vi "Set acquisition mode.vi"(8 "Error In":errorcluster, 9 "Synchronous acquisition":bool, 11 "Camera reference in":refnum<k24>) -> (0 "Error Out":errorcluster, 3 "Camera reference out":refnum<k24>)   [LabVIEW 2017]
uses:
  C:/Program Files/National Instruments/LabVIEW 2017/instr.lib/IDS/ueye.NET/uEyeDotNet.dll
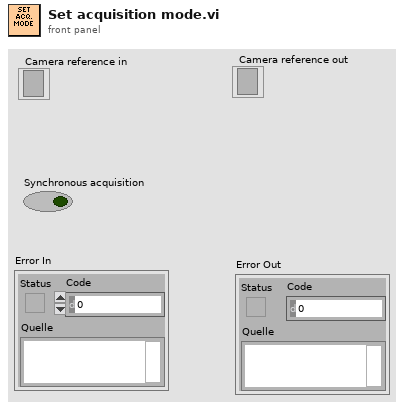
[diagram p1: front panel]
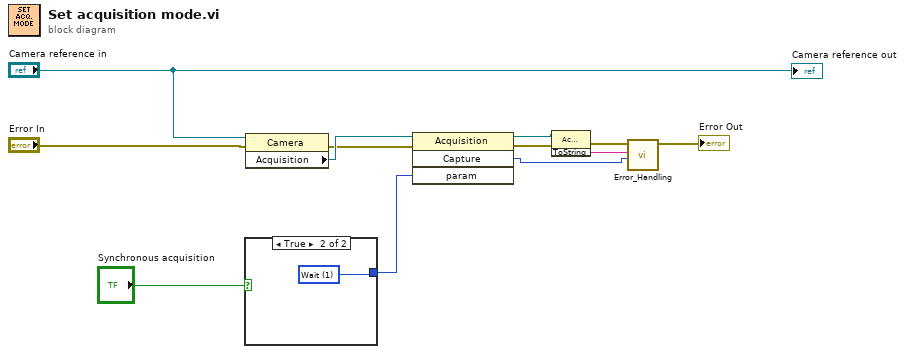
[diagram p0: block diagram]
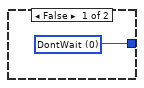
[diagram p2: hidden frame]
diagram:
  n1 = case shown="True" "Synchronous acquisition" {
    tunnel: [w13 w14] -> w11
    frame False {
      w13 = 0 items=["DontWait"=0, "Wait"=1, "Force"=16384] ("param")
    }
    frame True {
      w14 = 1 items=["DontWait"=0, "Wait"=1, "Force"=16384] ("param")
    }
  }
  n2 = property class="Camera"(reference="Camera reference in", error in="Error In") -> (error out=w9:errorcluster, "Acquisition"=w12:refnum<k24>)  [unwired: 1 out]
  n3 = invoke class="Acquisition" method="Capture"(reference=w12, error in=w9, "param"=w11) -> (reference out=w3:refnum<k24>, error out=w4:errorcluster, "Capture"=w2:i32)  [unwired: 1 in, 1 out]
  n4 = invoke class="Acquisition" method="ToString"(reference=w3, error in=w4) -> (error out=w7:errorcluster, "ToString"=w6:string)  [unwired: 1 in, 1 out]
  n5 = call <instrlib>:"Error_Handling.vi"("Error Code"=w2, "Error String"=w6, "Error In"=w7) -> ("Error Out"=→"Error Out":errorcluster)  [unwired: 8 in]
  "Camera reference out" <- "Camera reference in"
